vi "Delete Gradient 32f.vi"(8 "Error In":errorcluster, 11 "Gradient Object":T1 {"Z"."Dimension"."Width" min=1; "Z"."Dimension"."Height" min=1; "Z"."Dimension"."Depth" min=1; "Y"."Dimension"."Width" min=1; "Y"."Dimension"."Height" min=1; "Y"."Dimension"."Depth" min=1; "X"."Dimension"."Width" min=1; "X"."Dimension"."Height" min=1; "X"."Dimension"."Depth" min=1}) -> (0 "Error Out":errorcluster)   [LabVIEW 2012, in "OpenCLV x64.lvlib"]
doc: "Deletes the Gradient Object and all associated memory."
uses:
  OpenCLV x64.lvlib
  Controls/Gradient Object.ctl
  Controls/Program Handle.ctl
  Controls/Device ID.ctl
  Controls/Memory Object.ctl
  Controls/Memory ID.ctl
  User Controls/Array Dimensions.ctl
  Controls/Memory Type.ctl
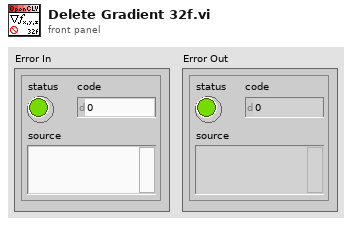
[diagram p1: front panel]
types:
  T1 = typedef "OpenCLV x64.lvlib/Gradient Object.ctl" = cluster{"Program Handle":T2, "Device Out":T3, "X":T4, "Y":T4, "Z":T4}
  T2 = typedef "OpenCLV x64.lvlib/Program Handle.ctl" = u64
  T3 = typedef "OpenCLV x64.lvlib/Device ID.ctl" = u64
  T4 = typedef "OpenCLV x64.lvlib/Memory Object.ctl" = cluster{"Device ID":T3, "Memeroy ID":T5, "Dimension":T6, "Memory Type":T7}
  T5 = typedef "OpenCLV x64.lvlib/Memory ID.ctl" = u64
  T6 = typedef "Array Dimensions.ctl" = cluster{"Depth":u64, "Height":u64, "Width":u64}
  T7 = typedef "OpenCLV x64.lvlib/Memory Type.ctl" = enum16{"32f", "u8", "i8", "u16", "i16", "u32", "i32", "64f"}
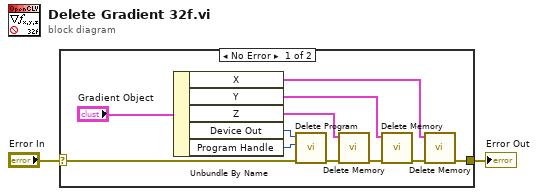
[diagram p0: block diagram]
diagram:
  n1 = case shown="No Error" "Error In" {
    selector: "Error In" -> [w11 w14]
    tunnel: [w7 w14] -> w1
    frame No Error {
      n2 = Unbundle By Name("Gradient Object") -> ("X"=w3:T4, "Y"=w4:T4, "Z"=w5:T4, "Device Out"=w6:T3, "Program Handle"=w12:T2)
      n3 = call "Delete Program.vi"("Error In"=w11, "Program In"=w12, "Device ID"=w6) -> ("Error Out"=w10:errorcluster)  [unwired: 8 in]
      n4 = call "Delete Memory.vi"("Error In"=w10, "Memory Object In"=w5) -> ("Error Out"=w9:errorcluster)  [unwired: 8 in, 1 out]
      n5 = call "Delete Memory.vi"("Error In"=w9, "Memory Object In"=w4) -> ("Error Out"=w8:errorcluster)  [unwired: 8 in, 1 out]
      n6 = call "Delete Memory.vi"("Error In"=w8, "Memory Object In"=w3) -> ("Error Out"=w7:errorcluster)  [unwired: 8 in, 1 out]
    }
    frame Error {
    }
  }
  "Error Out" <- w1
